vi "Dual Fan Test.vi"() -> ()   [LabVIEW 2012]
uses:
  Dual Controller/Dual Fan/Dual Fan.lvclass
  <vilib>/ActorFramework/Message Queue/Message Queue.lvclass/Message Queue.ctl
  <vilib>/ActorFramework/Message Enqueuer/Message Enqueuer.lvclass/Message Enqueuer.ctl
  <vilib>/ActorFramework/Message Enqueuer/Enqueue.vi
  <vilib>/ActorFramework/Message Priority Queue/Priority Enqueue.vi
  <vilib>/ActorFramework/Stop Msg/Stop Msg.lvclass
  Dual Controller/Power Off Msg/Power Off Msg.lvclass
  Dual Controller/Power On Msg/Power On Msg.lvclass
  <vilib>/ActorFramework/Actor/Actor.lvclass
  <vilib>/ActorFramework/Message Queue/Message Queue.lvclass
panel:
  in  "Fan State":bool
  in  "stop":bool
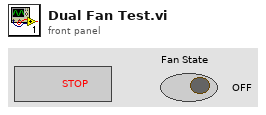
[diagram p1: front panel]
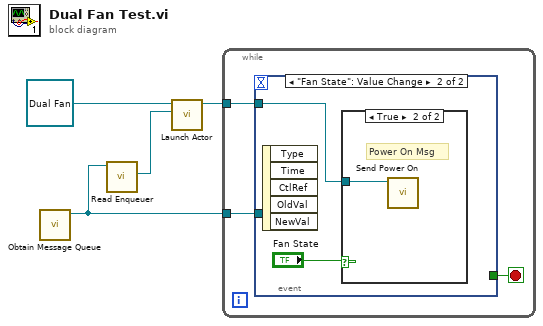
[diagram p0: block diagram]
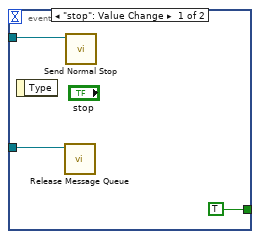
[diagram p2: hidden frame]
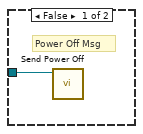
[diagram p3: hidden frame]
diagram:
  n1 = call <vilib>:"Obtain Message Queue.vi"() -> ("Message Queue"=w3:refnum<class "Message Queue.lvclass">)  [unwired: 10 in, 1 out]
  n2 = call <vilib>:"Read Enqueuer.vi"("Message Queue"=w3) -> ("Message Enqueuer"=w1:refnum<class "Message Enqueuer.lvclass">)  [unwired: 10 in]
  n3 = call <vilib>:"Launch Actor.vi"("Actor-to-Caller Enqueuer"=w1, "Actor"=refnum<class "Dual Fan.lvclass"> refnum ("Dual Fan.lvlib:Dual Fan.lvclass")) -> ("Caller-To-Actor Enqueuer"=w2:refnum<class "Message Enqueuer.lvclass">)  [unwired: 8 in, 1 out]
  n4 = while {
    tunnel: w3 -> [w7]
    tunnel: w2 -> [w6]
    stop <- w5 stop-if-true
    n5 = event shown="[1] \"Fan State\": Value Change" {
      selector: _ -> [_ _]
      dyn-events: _ -> [_ _]
      timeout: _ -> [_ _]
      tunnel: w6 -> [w10 w11]
      tunnel: w7 -> [w9 _]
      tunnel: [TRUE _] -> w5
      event "stop": Value Change {
        n6 = event-data() -> ()  [unwired: 1 in, 1 out]
        n7 = call <vilib>:"Release Message Queue.vi"("Message Queue"=w9) -> ()  [unwired: 9 in, 2 out]
        n8 = call <vilib>:"Send Normal Stop.vi"("Message Enqueuer"=w10) -> ()  [unwired: 10 in, 1 out]
      }
      event "Fan State": Value Change {
        n9 = event-data() -> ()  [unwired: 1 in, 5 out]
        n10 = case shown="True" "Fan State" {
          tunnel: w11 -> [w13 w14]
          frame False {
            # "Power Off Msg"
            n11 = call "Send Power Off.vi"("enqueuer"=w13) -> ()  [unwired: 10 in, 1 out]
          }
          frame True {
            # "Power On Msg"
            n12 = call "Send Power On.vi"("enqueuer"=w14) -> ()  [unwired: 10 in, 1 out]
          }
        }
      }
    }
  }
